vi "CountMatches1D.vi"(11 "Array":dbl[](array[numeric])) -> (0 "Result":dbl[](array[numeric]), 3 "History":dbl[](array[numeric]))   [LabVIEW 2023]
panel:
  out "Numeric":i32
  out "idx":dbl
  out "Number":dbl
  out "Result tmp":dbl[](array[numeric])
  out "History tmp":dbl[](array[numeric])
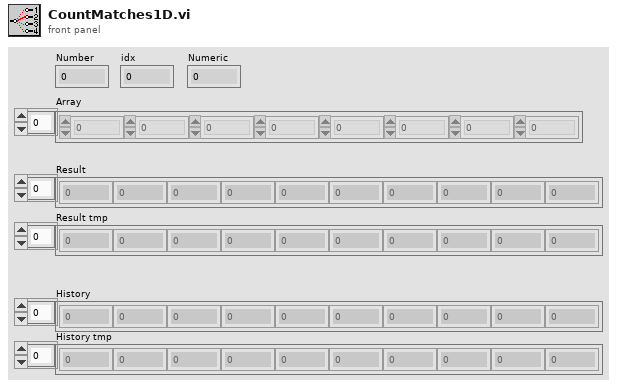
[diagram p1: front panel]
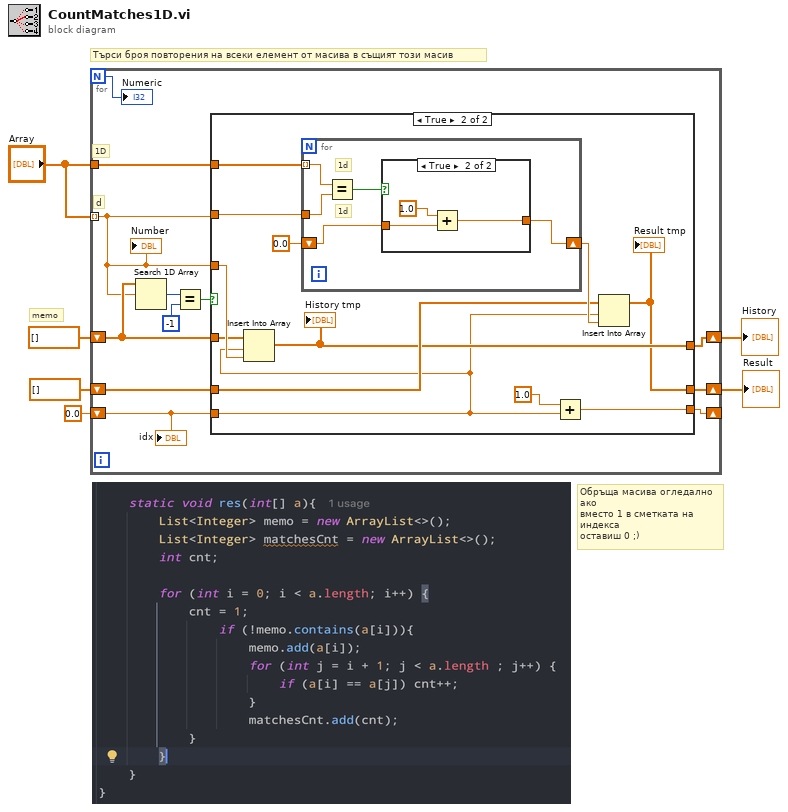
[diagram p0: block diagram]
diagram:
  # "memo"
  # "Търси броя повторения на всеки елемент от масива в същият този масив"
  # "Обръща масива огледално ако\nвместо 1 в сметката на индекса\nоставиш 0 ;)"
  n1 = for {
    N -> [w7]
    tunnel: "Array" -> [w15]
    tunnel: "Array" -> [w10] mode=indexing
    shift-right: [w13] -> w4
    shift-left: dbl[] [] -> [w14]
    shift-right: [w12] -> w2
    shift-left: dbl[] [] -> [w11]
    shift-right: [w9] -> _
    shift-left: 0.0 -> [w8]
    # "d"
    # "1D"
    n2 = Search 1D Array(1D array=w14, element=w10) -> (index of element=w18:i32)  [unwired: 1 in]
    n3 = Equal?(x=w18, y=-1) -> (x = y?=w16:bool)
    n4 = case shown="True" w16 {
      tunnel: w15 -> [_ w33]
      tunnel: w10 -> [_ w32]
      tunnel: w10 -> [_ w30]
      tunnel: w14 -> [w21 w29]
      tunnel: [w21 w26] -> w13
      tunnel: [w20 w25] -> w12
      tunnel: w11 -> [w20 w27]
      tunnel: w8 -> [w19 w22]
      tunnel: [w19 w23] -> w9
      frame False {
      }
      frame True {
        n5 = Insert Into Array(array=w29, index=w22, new element=w30) -> (w26:dbl[])
        "History tmp" <- w26
        n6 = for {
          tunnel: w33 -> [w38] mode=indexing
          tunnel: w32 -> [w37]
          shift-right: [w35] -> w28
          shift-left: 0.0 -> [w34]
          # "1d"
          # "1d"
          n7 = Equal?(x=w38, y=w37) -> (x = y?=w36:bool)
          n8 = case shown="True" w36 {
            tunnel: [w39 w41] -> w35
            tunnel: w34 -> [w39 w40]
            frame False {
            }
            frame True {
              n9 = Add(x=1.0, y=w40) -> (x+y=w41:dbl)
            }
          }
        }
        n10 = Add(x=1.0, y=w22) -> (x+y=w23:dbl)
        n11 = Insert Into Array(array=w27, index=w22, new element=w28) -> (w25:dbl[])
        "Result tmp" <- w25
      }
    }
    "Number" <- w10
    "idx" <- w8
    "Numeric" <- w7
  }
  "History" <- w4
  "Result" <- w2
